vi "C37 Poll PDC With Data Waiting.vi"(8 "error in (no error)":errorcluster, 10 "Poll Timeout [5 ms]":i32=5, 11 "Pseudo PDC ID":i32=5) -> (0 "error out":errorcluster, 3 "Data?":bool)   [LabVIEW 2013, in "C37118-DLL.lvlib"]
uses:
  C37118-DLL.lvlib
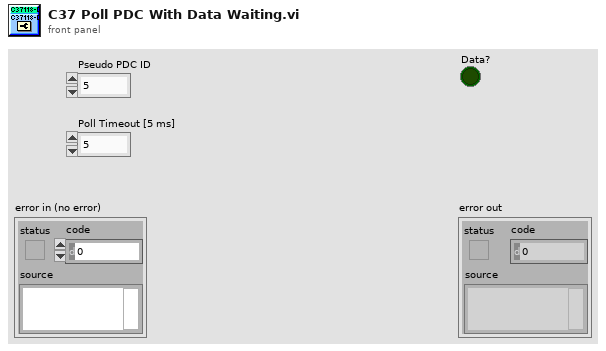
[diagram p1: front panel]
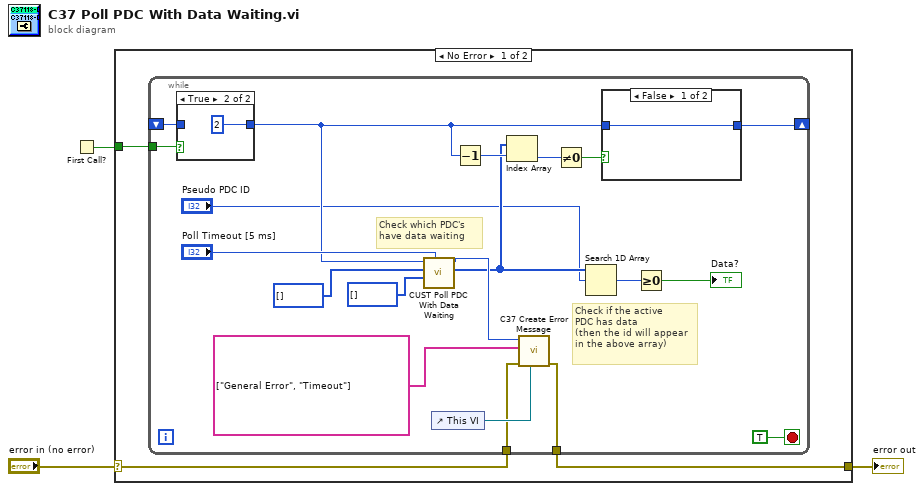
[diagram p0: block diagram]
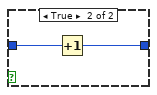
[diagram p2: hidden frame]
diagram:
  n1 = First Call?() -> (First Call?: T/F=w1:bool)
  n2 = case shown="No Error" "error in (no error)" {
    selector: "error in (no error)" -> [w6 w32]
    tunnel: [w5 w32] -> w3
    tunnel: w1 -> [w4 _]
    frame No Error {
      n3 = while {
        tunnel: w6 -> [w25]
        tunnel: [w24] -> w5
        tunnel: w4 -> [w17]
        shift-right: [w11] -> _
        shift-left: _ -> [w16]
        stop <- TRUE stop-if-true
        # "Check if the active\nPDC has data\n(then the id will appear\nin the above array)"
        # "Check which PDC's\nhave data waiting"
        n4 = case shown="True" w17 {
          tunnel: [w30 2 ("pseudoPdcIdArrayLength")] -> w12
          tunnel: w16 -> [w30 _]
          frame False {
          }
          frame True {
          }
        }
        n5 = call "CUST Poll PDC With Data Waiting.vi"("pollTimeoutMs"="Poll Timeout [5 ms]", "outNumPdcWithData"=i32[] [], "outPseudoPdcIdArr"=i32[] [], "pseudoPdcIdArrayLength"=w12) -> ("outPseudoPdcIdArr out"=w10:i32[], "function return"=w22:i32)  [unwired: 5 in, 1 out]
        n6 = control-ref of="This VI"() -> (w26:refnum<vi>)
        n7 = Decrement(x=w12) -> (x-1=w15:i32)
        n8 = Index Array(array=w10, index=w15) -> (element=w14:i32)
        n9 = call "C37 Create Error Message.vi"("VI Reference"=w26, "error in (no error)"=w25, "Error Messages"=string[] ["General Error", "Timeout"], "function return"=w22) -> ("error out"=w24:errorcluster)  [unwired: 7 in]
        n10 = Not Equal To 0?(x=w14) -> (x != 0?=w13:bool)
        n11 = Search 1D Array(1D array=w10, element="Pseudo PDC ID") -> (index of element=w8:i32)  [unwired: 1 in]
        n12 = case shown="False" w13 {
          tunnel: w12 -> [w27 w29]
          tunnel: [w27 w28] -> w11
          frame False {
          }
          frame True {
            n13 = Increment(x=w29) -> (x+1=w28:i32)
          }
        }
        n14 = Greater Or Equal To 0?(x=w8) -> (x >= 0?=→"Data?":bool)
      }
    }
    frame Error {
    }
  }
  "error out" <- w3
